vi "Stream Four Probe Asynchronous.vi"(10 "Error Stream gRPCid":T1, 11 "gRPCid":T1) -> ()   [LabVIEW 2019]
uses:
  labview-grpc-query-server/VIs/MeasurementServer_gRPCid.ctl
  Global Operations.ctl
  labview-grpc-query-server/VIs/labview-grpc-measurement-server.lvlib
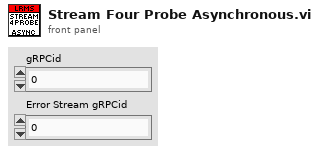
[diagram p1: front panel]
types:
  T1 = typedef "labview-grpc-measurement-server.lvlib/MeasurementServer_gRPCid.ctl" = u64
  T2 = typedef "Global Operations.ctl" = enum16{"Get", "Set"}
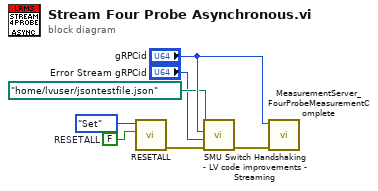
[diagram p0: block diagram]
diagram:
  w5 = FALSE  # RESETALL
  n1 = call "RESETALL.vi"("RESETALL"=w5, "Operation"=Global_Operations."Set") -> ("error out"=w3:errorcluster)  [unwired: 8 in, 1 out]
  n2 = call "SMU Switch Handshaking - LV code improvements - Streaming.vi"("error in"=w3, "Error Stream gRPCid"="Error Stream gRPCid", "gRPCid"="gRPCid", "file path (use dialog)"=path "/home/lvuser/jsontestfile.json") -> ("error out"=w1:errorcluster)  [unwired: 6 in, 1 out]
  n3 = call "MeasurementServer_FourProbeMeasurementComplete.vi"("gRPCid"="gRPCid", "error in (no error)"=w1) -> ()  [unwired: 8 in, 1 out]
